vi "FedorEnterZeros.vi"(8 "error in (no error)":errorcluster, 10 "DAQmx Device Name":tag="6251") -> (0 "error out":errorcluster)   [LabVIEW 2015]
uses:
  <vilib>/DAQmx/write.llb/DAQmx Write (Digital U8 1Chan 1Samp).vi
  <vilib>/DAQmx/create/channels.llb/DAQmx Create Channel (DO-Digital Output).vi
  <vilib>/DAQmx/miscellaneous.llb/DAQmx Fill In Error Info.vi
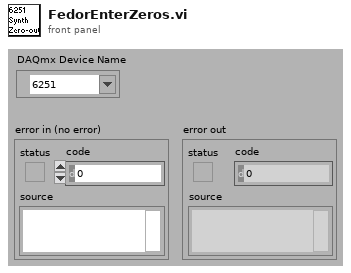
[diagram p1: front panel]
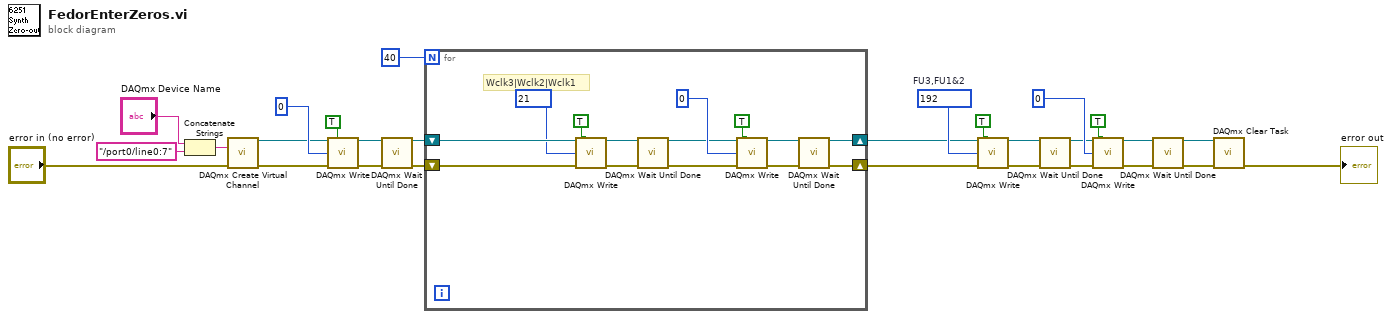
[diagram p0: block diagram]
diagram:
  w15 = u8 192  # FU3,FU1&2
  n1 = Concatenate Strings("DAQmx Device Name", "/port0/line0:7") -> (w4:string)
  n2 = call-poly <vilib>:"DAQmx Create Virtual Channel.vi"("lines"=w4, "error in"="error in (no error)") -> ("task out"=w21:refnum<k21>, "error out"=w27:errorcluster)  [unwired: 3 in, 9 out]
  n3 = call-poly <vilib>:"DAQmx Write.vi"("task/channels in"=w21, "auto start"=TRUE, "data"=u8 0, "error in"=w27) -> ("task out"=w20:refnum<k21>, "error out"=w26:errorcluster)  [unwired: 10 out]
  n4 = call <vilib>:"DAQmx Wait Until Done.vi"("task/channels in"=w20, "error in"=w26) -> ("task out"=w19:refnum<k21>, "error out"=w22:errorcluster)  [unwired: 1 in, 11 out]
  n5 = for {
    N: 40 -> [_]
    shift-right: [w29] -> w5
    shift-left: w22 -> [w42]
    shift-right: [w30] -> w6
    shift-left: w19 -> [w41]
    # "Wclk3|Wclk2|Wclk1"
    n6 = call-poly <vilib>:"DAQmx Write.vi"("task/channels in"=w41, "auto start"=TRUE, "data"=21 ("Waveform"), "error in"=w42) -> ("task out"=w38:refnum<k21>, "error out"=w40:errorcluster)  [unwired: 10 out]
    n7 = call <vilib>:"DAQmx Wait Until Done.vi"("task/channels in"=w38, "error in"=w40) -> ("task out"=w32:refnum<k21>, "error out"=w31:errorcluster)  [unwired: 1 in, 11 out]
    n8 = call-poly <vilib>:"DAQmx Write.vi"("task/channels in"=w32, "auto start"=TRUE, "data"=u8 0 ("Waveform"), "error in"=w31) -> ("task out"=w34:refnum<k21>, "error out"=w36:errorcluster)  [unwired: 10 out]
    n9 = call <vilib>:"DAQmx Wait Until Done.vi"("task/channels in"=w34, "error in"=w36) -> ("task out"=w30:refnum<k21>, "error out"=w29:errorcluster)  [unwired: 1 in, 11 out]
  }
  n10 = call-poly <vilib>:"DAQmx Write.vi"("task/channels in"=w6, "auto start"=TRUE, "data"=w15, "error in"=w5) -> ("task out"=w16:refnum<k21>, "error out"=w18:errorcluster)  [unwired: 10 out]
  n11 = call <vilib>:"DAQmx Wait Until Done.vi"("task/channels in"=w16, "error in"=w18) -> ("task out"=w10:refnum<k21>, "error out"=w9:errorcluster)  [unwired: 1 in, 11 out]
  n12 = call-poly <vilib>:"DAQmx Write.vi"("task/channels in"=w10, "auto start"=TRUE, "data"=u8 0 ("Waveform"), "error in"=w9) -> ("task out"=w12:refnum<k21>, "error out"=w14:errorcluster)  [unwired: 10 out]
  n13 = call <vilib>:"DAQmx Wait Until Done.vi"("task/channels in"=w12, "error in"=w14) -> ("task out"=w7:refnum<k21>, "error out"=w8:errorcluster)  [unwired: 1 in, 11 out]
  n14 = call <vilib>:"DAQmx Clear Task.vi"("task in"=w7, "error in"=w8) -> ("error out"=→"error out":errorcluster)  [unwired: 13 out]
